vi "Check Error.vi"(8 "error in (no error)":errorcluster, 11 "Error Code":i32) -> (0 "error out":errorcluster)   [LabVIEW 2021, in "CIF_NI_CIPC.lvlib"]
uses:
  CIF_NI_CIPC.lvlib
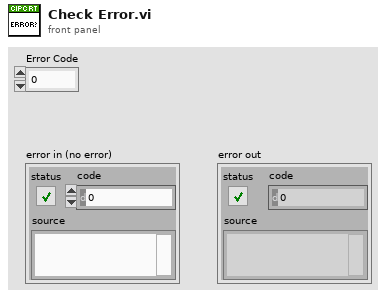
[diagram p1: front panel]
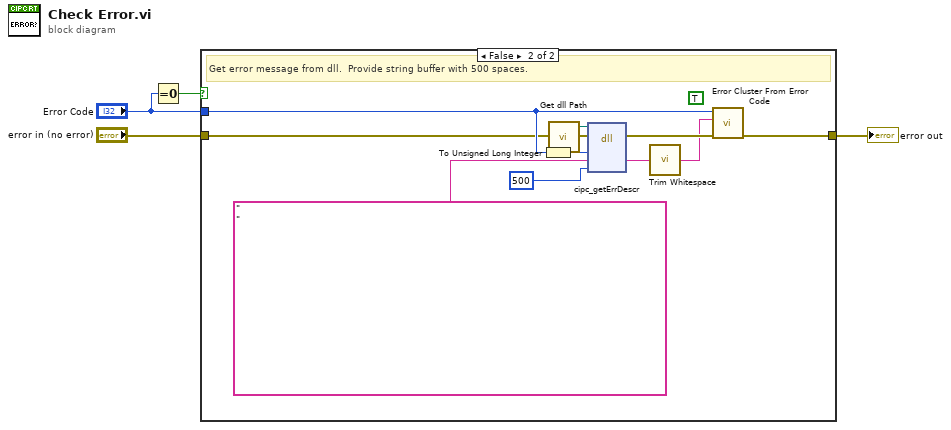
[diagram p0: block diagram]
diagram:
  n1 = Equal To 0?(x="Error Code") -> (x = 0?=w1:bool)
  n2 = case shown="False" w1 {
    tunnel: [w5 w15] -> w3
    tunnel: "error in (no error)" -> [w5 w12]
    tunnel: "Error Code" -> [_ w13]
    frame True {
    }
    frame False {
      (unwired) TRUE ("show call chain? (False)")
      # "Get error message from dll.  Provide string buffer with 500 spaces."
      n3 = To Unsigned Long Integer(number=w13) -> (unsigned 32bit integer=w8:u32)
      n4 = call "Get dll Path.vi"() -> ("appended path"=w6:path)  [unwired: 5 in]
      n5 = dll-call lib="libnicipc.*" fn="cipc_getErrDescr"(path in=w6, error in=w12, "err_code"=w8, "el_descr"="                                                                                                                                                                                                                                                                                                                                                                                                                                                                                                                    " ("string"), "el_descr_maxsize"=u32 500 ("dimension size")) -> (error out=w10:errorcluster, "el_descr"=w11:string)  [unwired: 4 in, 1 out]
      n6 = call <vilib>:"Trim Whitespace.vi"("string"=w11) -> ("trimmed string"=w7:string)  [unwired: 1 in]
      n7 = call <vilib>:"Error Cluster From Error Code.vi"("error in (no error)"=w10, "error message (\"\")"=w7, "error code (0)"=w13) -> ("error out"=w15:errorcluster)  [unwired: 6 in]
    }
  }
  "error out" <- w3
